vi "Shared Variable Server.vi"() -> ()   [LabVIEW 2020]
doc: "This VI hosts two shared variables that can be accessed by a variety of client VIs. Shared Variables are typically used for monitoring lossy data, like memory usage, temperature data, etc."
panel:
  in  "Stop":bool
  # "Overview: Demonstrates the use of Network-Published Shared Variables to provide monitoring data to a variety of client VIs.\nRequirements: Windows\nInstructions:\n1. Run this VI.\n2. Run each of the Shared Variable Client VIs in the project to see the different ways you can connect to shared variables. Note that any number of client VIs can run at the same time.\n3. Once you have stopped all the client VIs, click Stop to stop this VI."
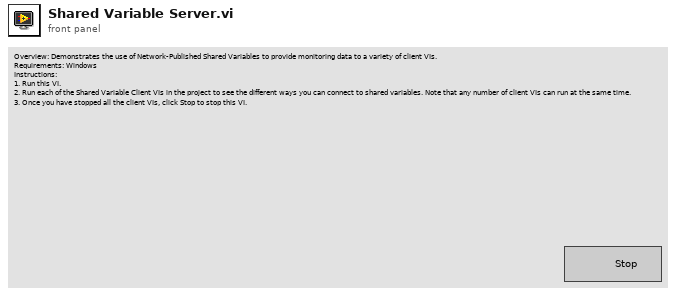
[diagram p1: front panel]
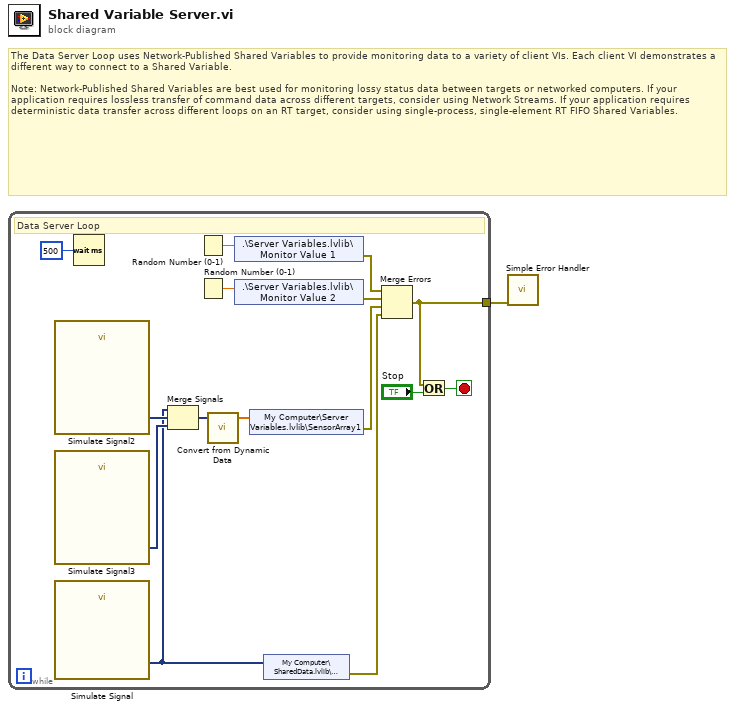
[diagram p0: block diagram]
diagram:
  # "The Data Server Loop uses Network-Published Shared Variables to provide monitoring data to a variety of client VIs. Each client VI demonstrates a different way to connect to a Shared Variable.\n\nNote: Network-Published Shared Variables are best used for monitoring lossy status data between targets or networked computers. If your application requires lossless transfer of command data across different targets, consider using Network Streams. If your application requires deterministic data transfer across different loops on an RT target, consider using single-process, single-element RT FIFO Shared Variables."
  n1 = while {
    tunnel: [w12] -> w1
    stop <- w15 stop-if-true
    # "Data Server Loop"
    n2 = call "Simulate Signal2"() -> ("Sine"=w5:dynamicdata)  [unwired: 14 in, 1 out]
    n3 = call "Simulate Signal3"() -> ("Sine"=w4:dynamicdata)  [unwired: 14 in, 1 out]
    n4 = call "Simulate Signal"() -> ("Sine"=w3:dynamicdata)  [unwired: 14 in, 1 out]
    n5 = Wait (ms)(milliseconds to wait=u32 500) -> ()  [unwired: 1 out]
    n6 = Merge Signals(w3, w5, w4) -> (w7:dynamicdata)
    n7 = Random Number (0-1)() -> (number: 0 to 1=w10:dbl)
    n8 = Random Number (0-1)() -> (number: 0 to 1=w9:dbl)
    n9 = call "Convert from Dynamic Data"("Dynamic Data Type"=w7) -> ("Array"=w8:dbl[])  [unwired: 3 in]
    n10 = shared-variable ".\\Server Variables.lvlib\\Monitor Value 1"(w10) -> (error out=w11:errorcluster)  [unwired: 1 in]
    n11 = shared-variable ".\\Server Variables.lvlib\\Monitor Value 2"(w9) -> (error out=w13:errorcluster)  [unwired: 1 in]
    n12 = shared-variable "My Computer\\Server Variables.lvlib\\SensorArray1"(w8) -> (error out=w6:errorcluster)  [unwired: 1 in]
    n13 = shared-variable "My Computer\\SharedData.lvlib\\Sensor1"(w3) -> (error out=w2:errorcluster)  [unwired: 1 in]
    n14 = Merge Errors(w11, w13, w6, w2) -> (w12:errorcluster)
    n15 = Or(x=w12, y="Stop") -> (x .or. y?=w15:bool)
  }
  n16 = call <vilib>:"Simple Error Handler.vi"("error in (no error)"=w1) -> ()  [unwired: 4 in, 5 out]
